vi "Alarma.vi"() -> ()   [LabVIEW 2020]
panel:
  out "Alarma 3":bool
  out "Alarma 2":bool
  out "Alarma 1":bool
  out "State  3":string
  out "State  2":string
  out "State  1":string
  in  "Minimo Temp.":u8(slide) scale=0.0..100.0
  in  "Maximo Temp.":u8(slide) scale=0.0..100.0
  in  "Termocupla  3":dbl(slide) scale=0.0..100.0
  in  "Termocupla  2":dbl(slide) scale=0.0..100.0
  in  "Termocupla1":dbl(slide) scale=0.0..100.0
  # "ALARMA INCENDIO"
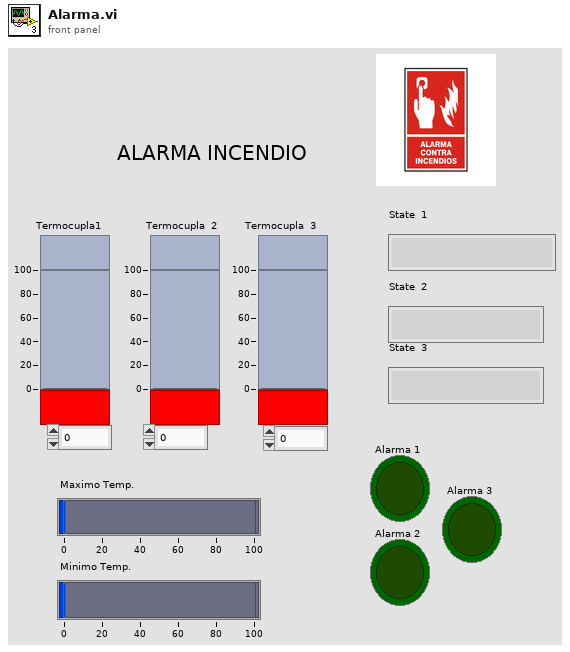
[diagram p1: front panel]
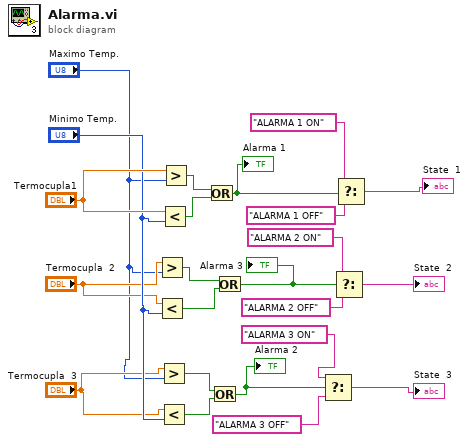
[diagram p0: block diagram]
diagram:
  n1 = Greater?(x="Termocupla  2", y="Maximo Temp.") -> (0:w21:bool)
  n2 = Less?(x="Termocupla  2", y="Minimo Temp.") -> (x < y?=w20:bool)
  n3 = Greater?(x="Termocupla  3", y="Maximo Temp.") -> (0:w19:bool)
  n4 = Less?(x="Termocupla  3", y="Minimo Temp.") -> (x < y?=w18:bool)
  n5 = Less?(x="Termocupla1", y="Minimo Temp.") -> (x < y?=w22:bool)
  n6 = Greater?(x="Termocupla1", y="Maximo Temp.") -> (0:w23:bool)
  n7 = Or(x=w23, y=w22) -> (x .or. y?=w17:bool)
  "Alarma 1" <- w17
  n8 = Or(x=w19, y=w18) -> (x .or. y?=w15:bool)
  "Alarma 2" <- w15
  n9 = Or(x=w21, y=w20) -> (x .or. y?=w14:bool)
  "Alarma 3" <- w14
  n10 = Select(t="ALARMA 3 ON", s=w15, f="ALARMA 3 OFF") -> (s? t:f=→"State  3":string)
  n11 = Select(t="ALARMA 2 ON", s=w14, f="ALARMA 2 OFF") -> (s? t:f=→"State  2":string)
  n12 = Select(t="ALARMA 1 ON", s=w17, f="ALARMA 1 OFF") -> (s? t:f=→"State  1":string)
